vi "Off-delay.vi"(1 "delay (ms)":u32, 2 "signal":bool) -> (0 "output":bool)   [LabVIEW 2009]
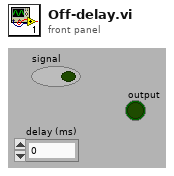
[diagram p1: front panel]
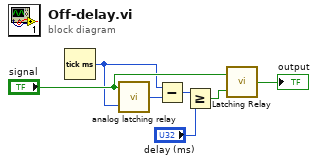
[diagram p0: block diagram]
diagram:
  n1 = Tick Count (ms)() -> (millisecond timer value=w2:u32)
  n2 = call "analog latching relay.vi"("value"=w2, "READ"="signal") -> ("out"=w1:u32)  [unwired: 1 in]
  n3 = Subtract(x=w2, y=w1) -> (x-y=w3:u32)
  n4 = Greater Or Equal?(x=w3, y="delay (ms)") -> (x >= y?=w5:bool)
  n5 = call "Latching Relay.vi"("Reset"=w5, "Trigger"="signal") -> ("output"=→"output":bool)
